vi "ImageFilter.vi"(6 "Chunk Size":u8, 9 "Filter\nIntensity":dbl, 10 "Filter\nCutoff":dbl, 11 "Array":dbl[][](array[numeric])) -> (3 "Array out":dbl[][](array[numeric]))   [LabVIEW 2021]
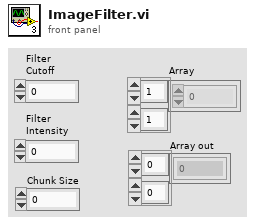
[diagram p1: front panel]
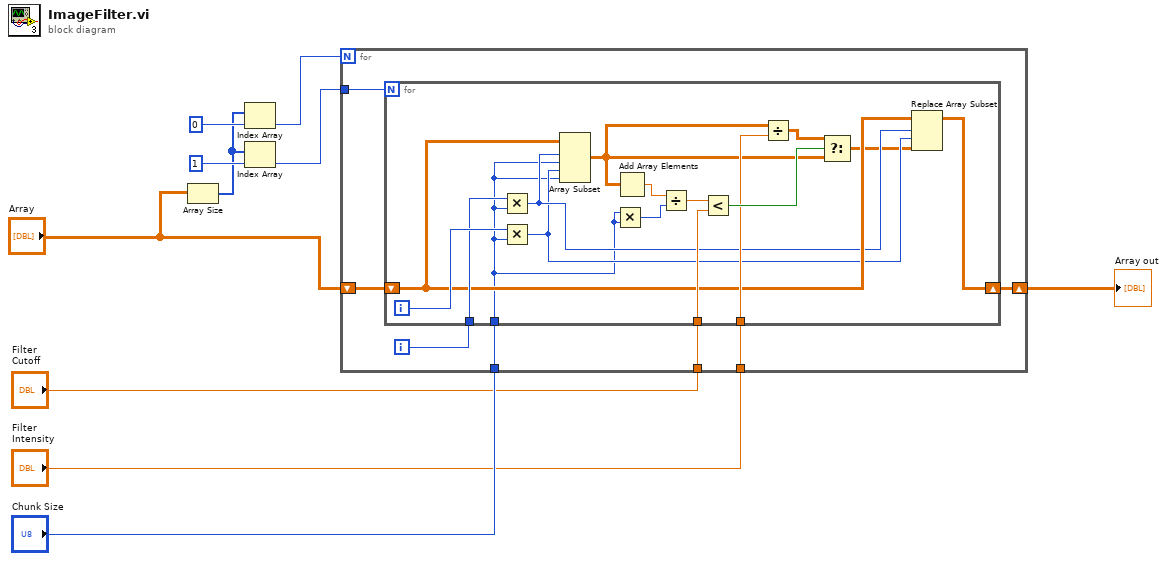
[diagram p0: block diagram]
diagram:
  n1 = Array Size(array="Array") -> (size(s)=w3:i32[])
  n2 = Index Array(array=w3, index=0) -> (element=w6:i32)
  n3 = Index Array(array=w3, index=1) -> (element=w7:i32)
  n4 = for {
    N: w6 -> [_]
    tunnel: w7 -> [w17]
    shift-right: [w15] -> w2
    shift-left: "Array" -> [w16]
    tunnel: "Filter\nCutoff" -> [w13]
    tunnel: "Filter\nIntensity" -> [w12]
    tunnel: "Chunk Size" -> [w11]
    i -> [w14]
    n5 = for {
      N: w17 -> [_]
      shift-right: [w20] -> w15
      shift-left: w16 -> [w24]
      tunnel: w14 -> [w32]
      tunnel: w13 -> [w30]
      tunnel: w12 -> [w27]
      tunnel: w11 -> [w18]
      i -> [w33]
      n6 = Multiply(x=w32, y=w18) -> (x*y=w23:i32)
      n7 = Multiply(x=w33, y=w18) -> (x*y=w22:i32)
      n8 = Array Subset(array=w24, index (row)=w23, length (row)=w18, index (col)=w22, length (col)=w18) -> (w26:dbl[][])
      n9 = Multiply(x=w18, y=w18) -> (x*y=w19:u8)
      n10 = Add Array Elements(numeric array=w26) -> (sum=w31:dbl)
      n11 = Divide(x=w31, y=w19) -> (x/y=w29:dbl)
      n12 = Less?(x=w29, y=w30) -> (x < y?=w28:bool)
      n13 = Divide(x=w26, y=w27) -> (x/y=w25:dbl[][])
      n14 = Select(t=w25, s=w28, f=w26) -> (s? t:f=w21:dbl[][])
      n15 = Replace Array Subset(array=w24, new element=w21, index (row)=w23, index (col)=w22) -> (w20:dbl[][])
    }
  }
  "Array out" <- w2
